vi "Testing.vi"() -> ()   [LabVIEW 2014]
panel:
  out "MonthDay":string
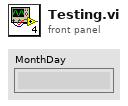
[diagram p1: front panel]
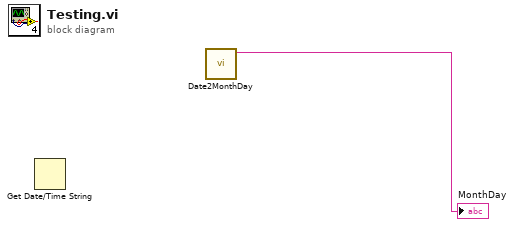
[diagram p0: block diagram]
diagram:
  n1 = Get Date/Time String() -> ()  [unwired: 3 in, 2 out]
  n2 = call "Date2MonthDay.vi"() -> ("MonthDay"=→"MonthDay":string)  [unwired: 10 in, 1 out]
